vi "Gather Results files specified in File.vi"() -> ()   [LabVIEW 2020]
panel:
  out "Current Path":path
  in  "New Data Directory":path
  out "Results files not found":path[](array[path])
  in  "File containing Results file paths":path
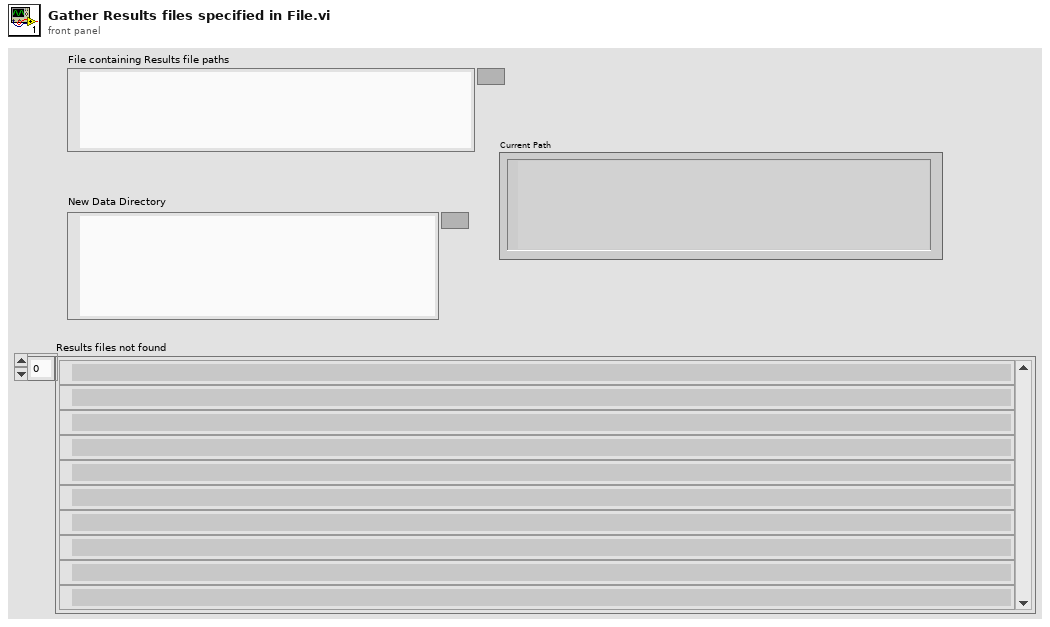
[diagram p1: front panel]
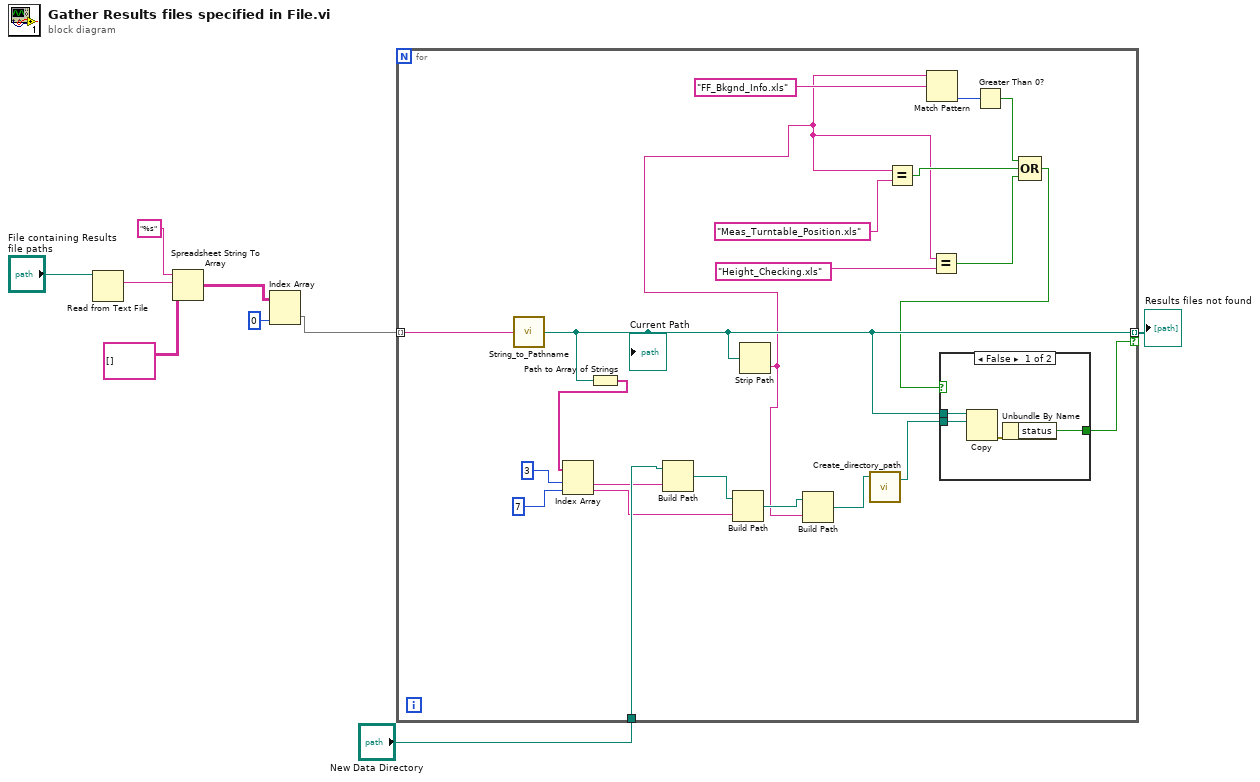
[diagram p0: block diagram]
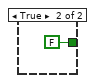
[diagram p2: hidden frame]
diagram:
  n1 = Read from Text File(file (use dialog)="File containing Results file paths") -> (text=w9:string)  [unwired: 3 in, 3 out]
  n2 = Spreadsheet String To Array(format string="%s", spreadsheet string=w9, array type (2D Dbl)=string[][] []) -> (array=w6:string[][])  [unwired: 1 in]
  n3 = Index Array(array=w6, index (col)=0 ("disabled index (col)")) -> (element=w3:string[])  [unwired: 1 in]
  n4 = for {
    tunnel: w3 -> [w31] mode=indexing
    tunnel: [w22] -> w2 mode=indexing if=w19
    tunnel: "New Data Directory" -> [w27]
    n5 = call "String_to_Pathname.vi"("Input String"=w31) -> ("path"=w22:path)
    "Current Path" <- w22
    n6 = Path to Array of Strings(0:w22) -> (2:w30:string[])  [unwired: 1 out]
    n7 = Index Array(array=w30, index #1=3 ("index"), index #2=7 ("index")) -> (element #1=w26:string, element #2=w24:string)
    n8 = Build Path(base path=w27, name or relative path=w26) -> (appended path=w25:path)
    n9 = Build Path(base path=w25, name or relative path=w24) -> (appended path=w23:path)
    n10 = Strip Path(path=w22) -> (name=w11:string)  [unwired: 1 out]
    n11 = Build Path(base path=w23, name or relative path=w11) -> (appended path=w21:path)
    n12 = call "Create_directory_path.vi"("Path name"=w21) -> ("Path name Out"=w20:path)  [unwired: 2 in, 1 out]
    n13 = Equal?(x=w11, y="Meas_Turntable_Position.xls") -> (x = y?=w15:bool)
    n14 = Match Pattern(string=w11, regular expression="FF_Bkgnd_Info.xls") -> (offset past match=w14:i32)  [unwired: 1 in, 3 out]
    n15 = Equal?(x=w11, y="Height_Checking.xls") -> (x = y?=w16:bool)
    n16 = Greater Than 0?(x=w14) -> (x > 0?=w13:bool)
    n17 = Compound Arithmetic op=OR(w13, w15, w16) -> (w10:bool)
    n18 = case shown="False" w10 {
      tunnel: w22 -> [w35 _]
      tunnel: w20 -> [w34 _]
      tunnel: [w32 FALSE ("status")] -> w19
      frame False {
        n19 = Copy(10:w34, 11:w35) -> (0:w33:errorcluster)  [unwired: 3 in, 2 out]
        n20 = Unbundle By Name(w33) -> ("status"=w32:bool)
      }
      frame True {
      }
    }
  }
  "Results files not found" <- w2
